vi "Insrument with scanner Front Panel.vi"(8 "error in (no error)":errorcluster, 11 "Class":refnum<class "Instrument with scanner.lvclass">) -> (0 "error out":errorcluster, 3 "Instrument with scanner out":refnum<class "Instrument with scanner.lvclass">)   [LabVIEW 2015]
uses:
  Instrument with scanner.lvclass
  Instrument with scanner Front Panel Data.ctl
panel:
  in  "Data":T1={"Channels to scan"=[], "Scan settling, s"=10.0}
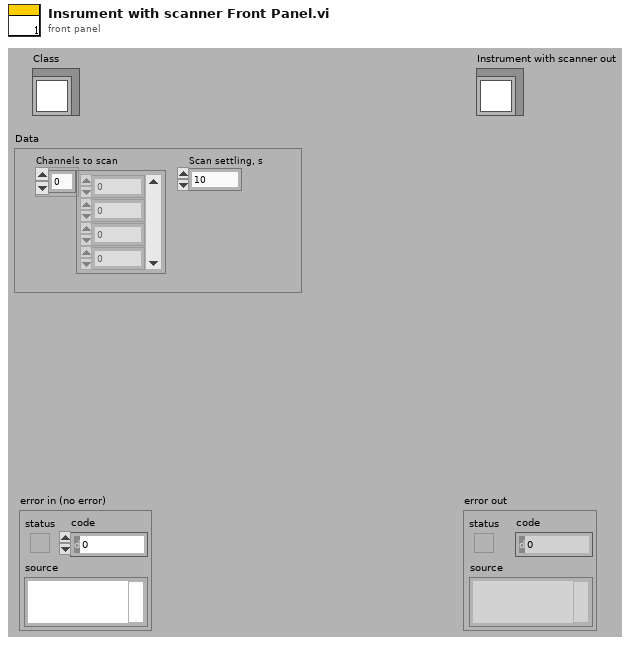
[diagram p1: front panel]
types:
  T1 = typedef "Instrument with scanner Front Panel Data.ctl" = cluster{"Channels to scan":i32[], "Scan settling, s":dbl}
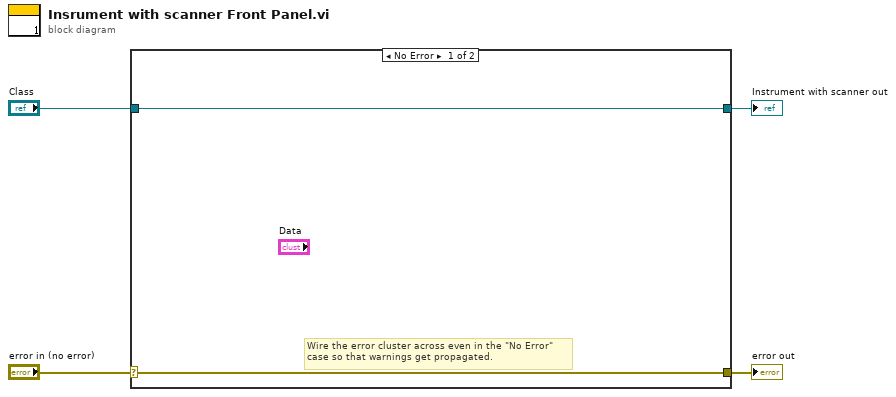
[diagram p0: block diagram]
diagram:
  n1 = case shown="No Error" "error in (no error)" {
    selector: "error in (no error)" -> [w5 w8]
    tunnel: [w5 w8] -> w3
    tunnel: [w6 w7] -> w1
    tunnel: "Class" -> [w6 w7]
    frame No Error {
      # "Wire the error cluster across even in the \"No Error\"\ncase so that warnings get propagated."
    }
    frame Error {
    }
  }
  "error out" <- w3
  "Instrument with scanner out" <- w1
